vi "CmdExe.Run Net Use.vi"(8 "error in":errorcluster, 9 "Show Cmd Window":bool=TRUE, 10 "Wait til Complete":bool=TRUE, 11 "Util Folder":path=path "C:/MTE/Startup") -> (0 "error out":errorcluster, 2 "StdOut":string[](array[string]), 3 "Cmd":string[](array[string]))   [LabVIEW 2019]
uses:
  <vilib>/KATE/Files/File Utils.lvlib
  <vilib>/KATE/Encryption/Encryption.lvlib
panel:
  out "Info":T1(array[cluster])
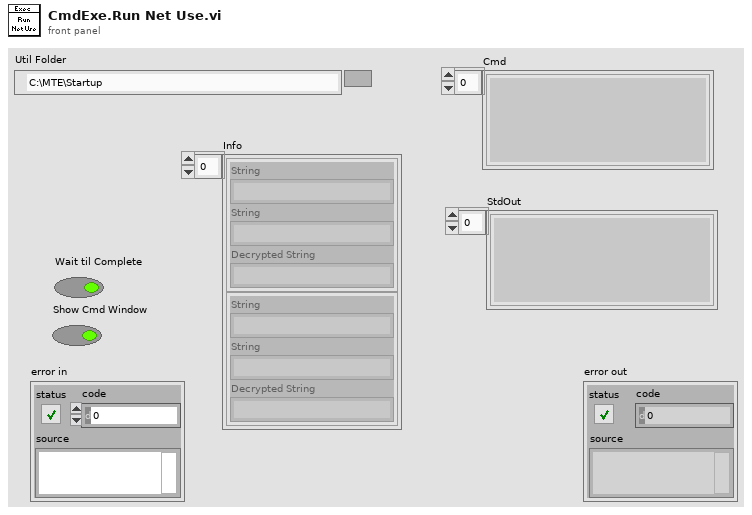
[diagram p1: front panel]
types:
  T1 = cluster{"String":string, "String":string, "Decrypted String":string}[]
  T2 = cluster{"String":string, "String":string, "Decrypted String":string}
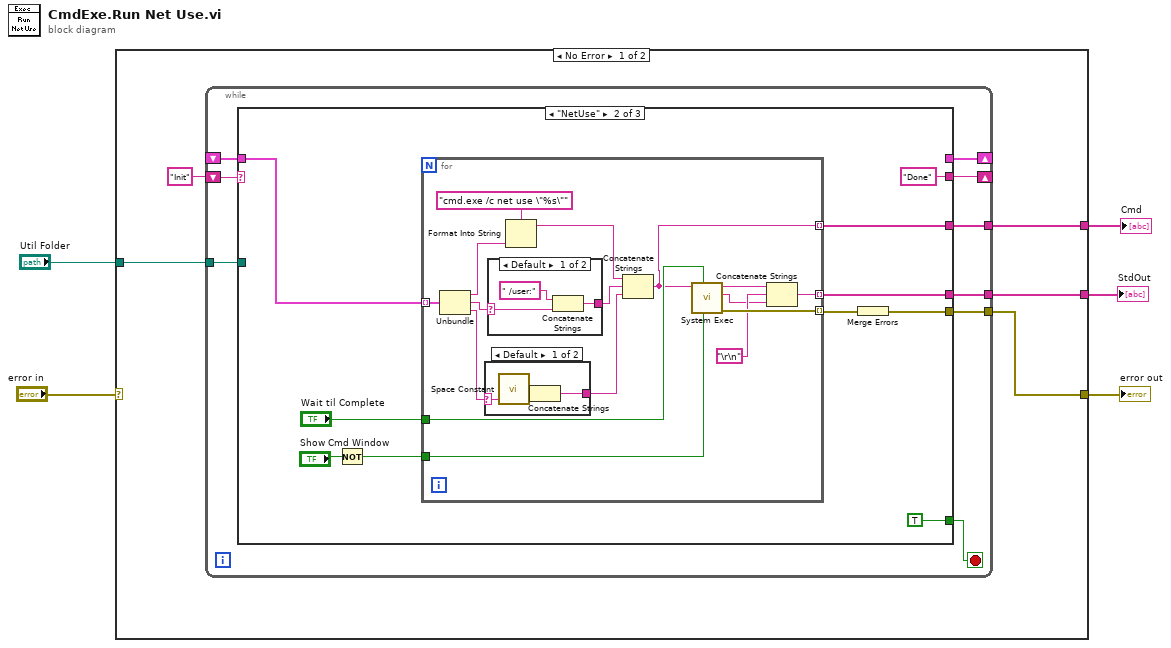
[diagram p0: block diagram]
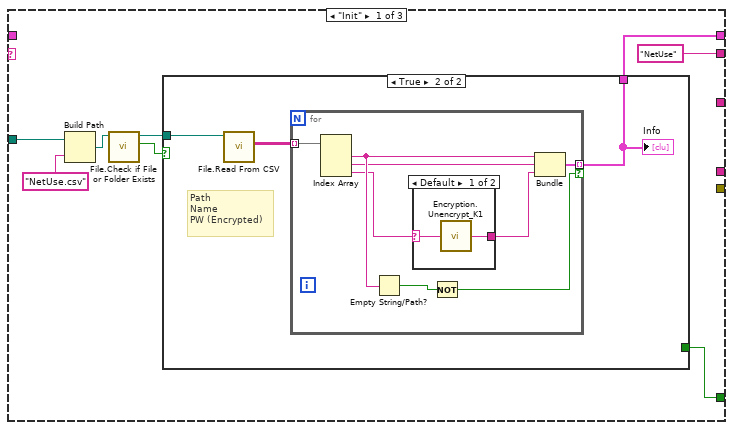
[diagram p2: hidden frame]
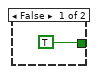
[diagram p3: hidden frame]
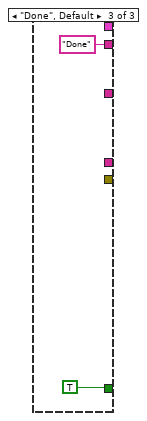
[diagram p7: hidden frame]
diagram:
  n1 = case shown="No Error" "error in" {
    selector: "error in" -> [_ w77]
    tunnel: "Util Folder" -> [w10 _]
    tunnel: [w8 _] -> w4
    tunnel: [w7 w77] -> w3
    tunnel: [w6 _] -> w1
    frame No Error {
      n2 = while {
        tunnel: w10 -> [w17]
        shift-right: [w14] -> _
        shift-left: "Init" -> [w19]
        shift-right: [w15] -> _
        shift-left: _ -> [w18]
        tunnel: [w13] -> w8
        tunnel: [w12] -> w7
        tunnel: [w11] -> w6
        stop <- w16 stop-if-true
        n3 = case shown="\"NetUse\"" w19 {
          tunnel: w18 -> [_ w48 _]
          tunnel: w17 -> [w27 _ _]
          tunnel: [w22 TRUE TRUE] -> w16
          tunnel: [w21 _ _] -> w15
          tunnel: ["NetUse" "Done" "Done"] -> w14
          tunnel: [_ w46 _] -> w13
          tunnel: [_ w44 _] -> w12
          tunnel: [_ w43 _] -> w11
          frame "Init" {
            n4 = Build Path(base path=w27, name or relative path="NetUse.csv") -> (appended path=w26:path)
            n5 = call <vilib>:"File.Check if File or Folder Exists.vi"("Path"=w26) -> ("Exists"=w24:bool, "Dup Path"=w23:path)  [unwired: 6 in, 3 out]
            n6 = case shown="True" w24 {
              tunnel: w23 -> [_ w31]
              tunnel: [TRUE _] -> w22
              tunnel: [_ w29] -> w21
              frame False {
              }
              frame True {
                # "Path\nName\nPW (Encrypted)"
                n7 = call <vilib>:"File.Read From CSV.vi"("File"=w31) -> ("Data"=w30:string[][])  [unwired: 8 in, 2 out]
                n8 = for {
                  tunnel: w30 -> [w39] mode=indexing
                  tunnel: [w36] -> w29 mode=indexing if=w32
                  n9 = Index Array(array=w39) -> (element #1=w38:string, element #2=w37:string, element #3=w34:string)  [unwired: 3 in]
                  n10 = Empty String/Path?(string/path=w38) -> (empty?=w33:bool)
                  n11 = case shown="Default" w34 {
                    selector: w34 -> [w40 w42]
                    tunnel: [w41 w42] -> w35
                    frame Default {
                      n12 = call <vilib>:"Encryption.Unencrypt_K1.vi"("Encrypted String"=w40) -> ("Decrypted String"=w41:string)
                    }
                    frame "" {
                    }
                  }
                  n13 = Not(x=w33) -> (.not. x?=w32:bool)
                  n14 = Bundle("String"=w38, "String"=w37, "Decrypted String"=w35) -> (w36:T2)  [unwired: 1 in]
                }
                "Info" <- w29
              }
            }
          }
          frame "NetUse" {
            n15 = Not(x="Show Cmd Window") -> (.not. x?=w50:bool)
            n16 = for {
              tunnel: [w68] -> w45 mode=indexing
              tunnel: w50 -> [w67]
              tunnel: "Wait til Complete" -> [w66]
              tunnel: w48 -> [w63] mode=indexing
              tunnel: [w58] -> w46 mode=indexing
              tunnel: [w53] -> w43 mode=indexing
              n17 = Unbundle(w63) -> ("String"=w62:string, "String"=w55:string, "Decrypted String"=w57:string)
              n18 = case shown="Default" w57 {
                selector: w57 -> [w73 _]
                tunnel: [w72 _] -> w56
                frame Default {
                  n19 = call <vilib>:"Space Constant.vi"() -> ("String"=w74:string)
                  n20 = Concatenate Strings(w74, w73) -> (w72:string)
                }
                frame "" {
                }
              }
              n21 = case shown="Default" w55 {
                selector: w55 -> [w71 _]
                tunnel: [w70 _] -> w54
                frame Default {
                  n22 = Concatenate Strings(" /user:", w71) -> (w70:string)
                }
                frame "" {
                }
              }
              n23 = Format Into String(format string="cmd.exe /c net use \"%s\"", w62) -> (resulting string=w64:string)  [unwired: 2 in, 1 out]
              n24 = Concatenate Strings(w64, w54, w56) -> (w53:string)
              n25 = call <vilib>:"System Exec.vi"("run minimized? (F)"=w67, "wait until completion? (T)"=w66, "command line"=w53) -> ("error out"=w68:errorcluster, "standard error"=w59:string, "standard output"=w61:string)  [unwired: 5 in, 1 out]
              n26 = Concatenate Strings(w61, "\r\n", w59) -> (w58:string)
            }
            n27 = Merge Errors(w45) -> (w44:errorcluster)
          }
          frame "Done", Default {
          }
        }
      }
    }
    frame Error {
    }
  }
  "error out" <- w3
  "StdOut" <- w4
  "Cmd" <- w1
